vi "SyncTime_HH.vi"() -> (0 "OverFlowConstant80Mhz(µs)":dbl)   [LabVIEW 2009]
panel:
  in  "Sync time (ns)":dbl=12.5
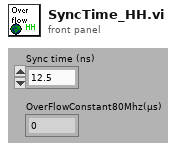
[diagram p1: front panel]
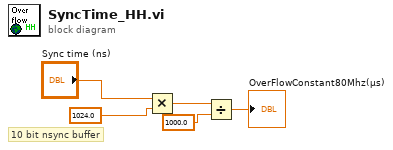
[diagram p0: block diagram]
diagram:
  # "10 bit nsync buffer"
  n1 = Multiply(x="Sync time (ns)", y=1024.0 ("x")) -> (x*y=w4:dbl)
  n2 = Divide(x=w4, y=1000.0) -> (x/y=→"OverFlowConstant80Mhz(µs)":dbl)
